vi "Rb_wavlength_lock.vi"(4 "Device":refnum<visa-resource-name>="GPIB0::10::INSTR", 6 "Settings":T2={"Module"=enum."WV Online TEC", "WV Online TEC"=23.169499999999484, "WV Online LD"=0.175, "WV Offline TEC"=29.51225, "WV Offline LD"=0.175, "WV Etalon TEC"=30.4, "HSRL Etalon TEC"=25.954, "HSRL TEC"=14.28699999999974, "HSRL LD"=0.16} {"HSRL LD" min=0.0 max=0.18 step=0.001 format="%.3p"; "HSRL TEC" min=14.0 max=28.0 step=0.1 format="%.3g"; "WV Offline LD" min=0.0 max=0.18 step=0.001 format="%.3p"; "WV Online LD" min=0.0 max=0.18 step=0.001 format="%.3p"; "HSRL Etalon TEC" format="%.2g"; "WV Etalon TEC" format="%.2g"; "WV Offline TEC" min=16.0 max=30.0 step=0.1 format="%.3g"; "WV Online TEC" min=14.0 max=28.0 step=0.1 format="%.3g"}, 7 "Lambda Set (nm)":dbl=828.198 format="%.5f", 8 "step_size":dbl=0.0005 format="%#_6p") -> (1 "Wavelength Lock":bool=TRUE, 2 "Lambda Read (nm)":dbl=828.197992104015 format="%.5f")   [LabVIEW 2012]
uses:
  <vilib>/DAQmx/write.llb/DAQmx Write (Digital 1D Bool NChan 1Samp 1Line).vi
  <vilib>/DAQmx/miscellaneous.llb/DAQmx Fill In Error Info.vi
  Shared Telescope WV DIAL Code/bristol/CLDevIFace.dll
panel:
  out "Readings":T1={"Pro8000"=TRUE, "WV OnLine TEC"=23.1755314, "WV Online TEC"=TRUE, "WV Online LD"=0.175443366, "WV Online LD"=TRUE, "WV Offline TEC"=29.5255375, "WV Offline TEC"=TRUE, "WV Offline LD"=0.175283208, "WV Offline LD"=TRUE, "WV EtalonTEC"=30.4229469, "WV Etalon TEC"=TRUE, "HSRL Etalon TEC"=25.9482574, "HSRL Etalon TEC"=TRUE, "HSRL TEC"=14.2977543, "HSRL TEC "=TRUE, "HSRL LD"=0.160093755, "HSRL LD"=TRUE} {"HSRL LD" format="%.3p"; "HSRL TEC" format="%.3g"; "WV Offline LD" format="%.3p"; "WV Online LD" format="%.3p"; "HSRL Etalon TEC" format="%.3g"; "WV EtalonTEC" format="%.3g"; "WV Offline TEC" format="%.3g"; "WV OnLine TEC" format="%.3g"}
  in  "Wavelength_lock_Tol":dbl=0.0001 format="%#_15g"
  out "WL_Difference":dbl=-7.895984936112654e-06 format="%#_3e"
  in  "Cancel lock":bool
  in  "Bristol In":i32=5
  out "Bristol Out":i32
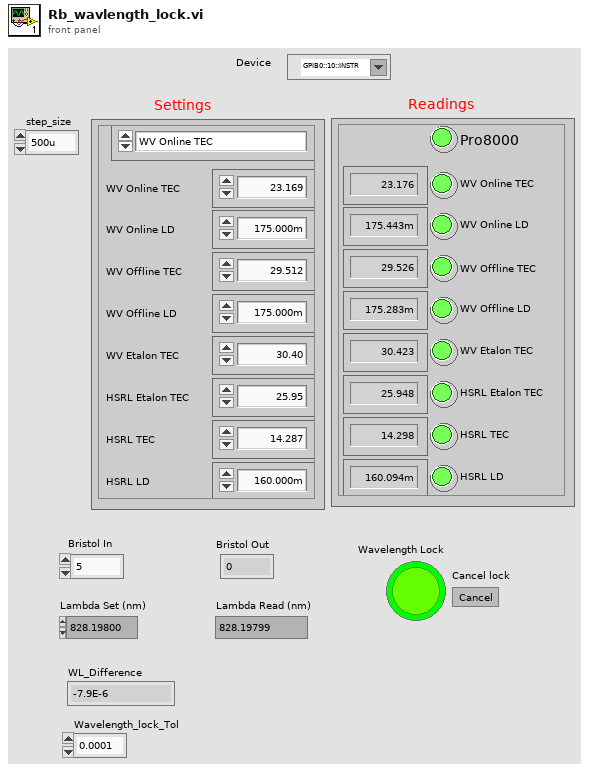
[diagram p1: front panel]
types:
  T1 = cluster{"Pro8000":bool, "WV OnLine TEC":dbl, "WV Online TEC":bool, "WV Online LD":dbl, "WV Online LD":bool, "WV Offline TEC":dbl, "WV Offline TEC":bool, "WV Offline LD":dbl, "WV Offline LD":bool, "WV EtalonTEC":dbl, "WV Etalon TEC":bool, "HSRL Etalon TEC":dbl, "HSRL Etalon TEC":bool, "HSRL TEC":dbl, "HSRL TEC ":bool, "HSRL LD":dbl, "HSRL LD":bool}
  T2 = cluster{"Module":enum16{"WV Online TEC", "WV Online LD", "WV Offline TEC", "WV Offline LD", "WV Etalon TEC", "HSRL Etalon TEC", "HSRL TEC", "HSRL LD"}, "WV Online TEC":dbl, "WV Online LD":dbl, "WV Offline TEC":dbl, "WV Offline LD":dbl, "WV Etalon TEC":dbl, "HSRL Etalon TEC":dbl, "HSRL TEC":dbl, "HSRL LD":dbl}
  T3 = enum16{"WV Online TEC", "WV Online LD", "WV Offline TEC", "WV Offline LD", "WV Etalon TEC", "HSRL Etalon TEC", "HSRL TEC", "HSRL LD"}
  T4 = enum16{"Open_TL", "Close_TL", "Verify_ID", "TEC_Sensor", "SET", "READ", "ON", "OFF", "Set_Limits", "Read_Limits", "Enable_Status", "Read_Status"}
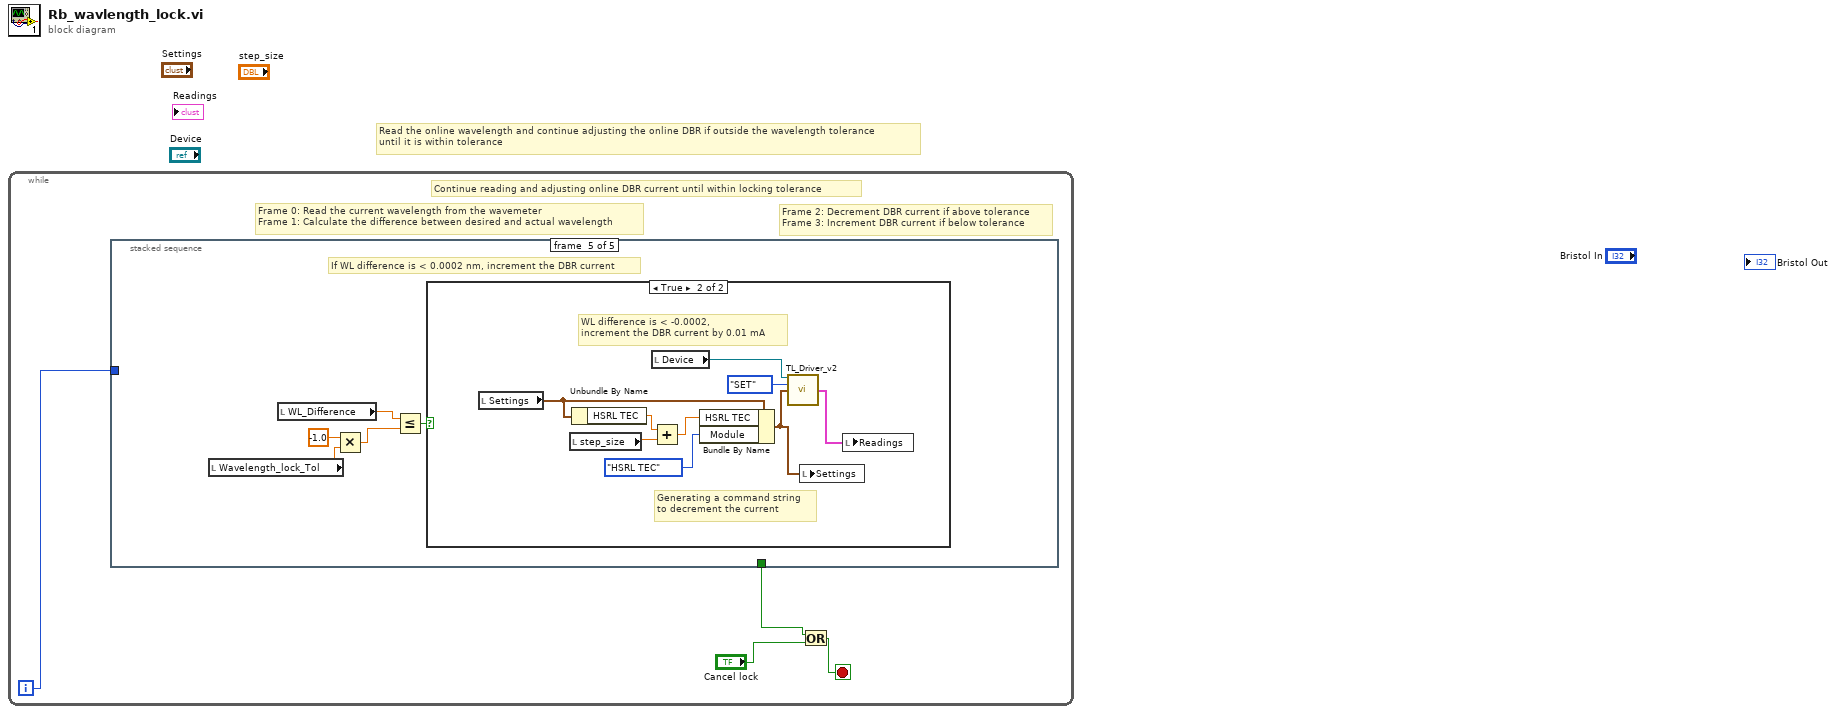
[diagram p0: block diagram]
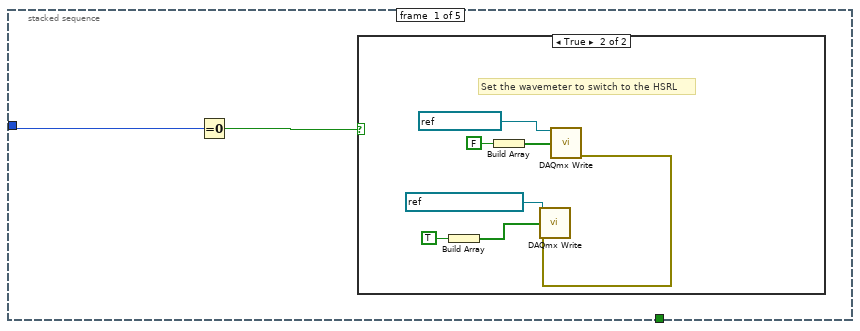
[diagram p2: hidden frame]
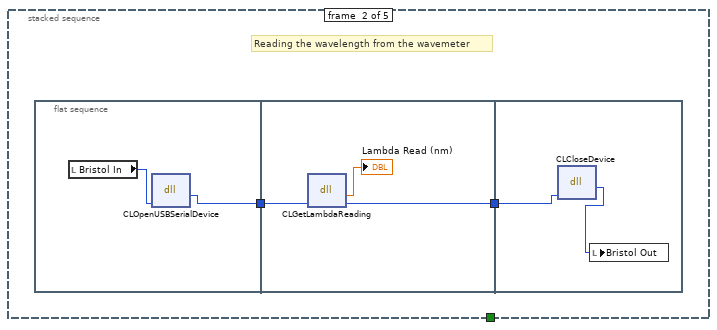
[diagram p4: hidden frame]
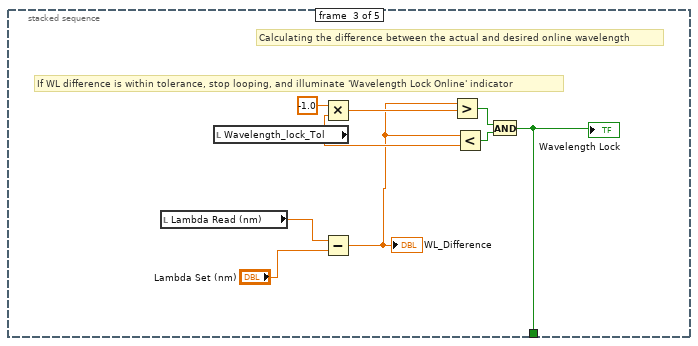
[diagram p5: hidden frame]
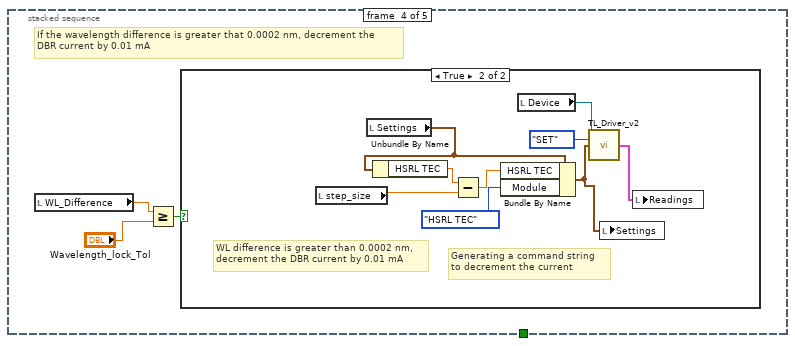
[diagram p6: hidden frame]
diagram:
  # "Read the online wavelength and continue adjusting the online DBR if outside the wavelength tolerance\nuntil it is within tolerance"
  n1 = while {
    i -> [w4]
    stop <- w1 stop-if-true
    # "Frame 2: Decrement DBR current if above tolerance\nFrame 3: Increment DBR current if below tolerance"
    # "Frame 0: Read the current wavelength from the wavemeter\nFrame 1: Calculate the difference between desired and actual wavelength"
    # "Continue reading and adjusting online DBR current until within locking tolerance"
    n2 = stacked-sequence {
      tunnel: w4 -> [w6 _ _ _ _]
      tunnel: [_ _ w23 _ _] -> w2
      frame #0 {
        n3 = Equal To 0?(x=w6) -> (x = 0?=w5:bool)
        n4 = case shown="True" w5 {
          frame False {
          }
          frame True {
            # "Set the wavemeter to switch to the HSRL"
            n5 = Build Array(TRUE ("Boolean")) -> (w8:bool[])
            n6 = Build Array(FALSE ("Boolean")) -> (w11:bool[])
            n7 = call-poly <vilib>:"DAQmx Write.vi"("task/channels in"=refnum<k21> "BristolWM", "data"=w11) -> ("error out"=w7:errorcluster)  [unwired: 11 in, 2 out]
            n8 = call-poly <vilib>:"DAQmx Write.vi"("task/channels in"=refnum<k21> "HSRL_WV_switch", "data"=w8, "error in"=w7) -> ()  [unwired: 10 in, 3 out]
          }
        }
      }
      frame #1 {
        # "Reading the wavelength from the wavemeter"
        n9 = flat-sequence {
          tunnel: [w16] -> w15
          tunnel: w15 -> [w19]
          tunnel: [w18] -> w14
          tunnel: w14 -> [w22]
          frame #0 {
            n10 = local read "Bristol In"() -> (w17:i32)
            n11 = dll-call lib="C:/Users/H2ODial/Desktop/Shared Telescope WV DIAL Code/bristol/CLDevIface.dll" fn="CLOpenUSBSerialDevice"("commPort"=w17) -> ("return type"=w16:i32)  [unwired: 4 in, 2 out]
          }
          frame #1 {
            n12 = dll-call lib="C:/Users/H2ODial/Desktop/Shared Telescope WV DIAL Code/bristol/CLDevIface.dll" fn="CLGetLambdaReading"("devHandle"=w19) -> ("return type"=→"Lambda Read (nm)":dbl, "devHandle"=w18:i32)  [unwired: 3 in, 2 out]
          }
          frame #2 {
            n13 = dll-call lib="C:/Users/H2ODial/Desktop/Shared Telescope WV DIAL Code/bristol/CLDevIface.dll" fn="CLCloseDevice"("commPort"=w22) -> ("return type"=w21:i32)  [unwired: 4 in, 2 out]
            n14 = local write "Bristol Out"(w21) -> ()
          }
        }
      }
      frame #2 {
        # "If WL difference is within tolerance, stop looping, and illuminate 'Wavelength Lock Online' indicator"
        # "Calculating the difference between the actual and desired online wavelength"
        n15 = local read "Lambda Read (nm)"() -> (w31:dbl)
        n16 = local read "Wavelength_lock_Tol"() -> (w28:dbl)
        n17 = Multiply(x=-1.0, y=w28) -> (x*y=w29:dbl)
        n18 = Subtract(x=w31, y="Lambda Set (nm)") -> (x-y=w24:dbl)
        "WL_Difference" <- w24
        n19 = Greater?(x=w24, y=w29) -> (0:w25:bool)
        n20 = Less?(x=w24, y=w28) -> (x < y?=w26:bool)
        n21 = And(x=w25, y=w26) -> (x .and. y?=w23:bool)
        "Wavelength Lock" <- w23
      }
      frame #3 {
        # "If the wavelength difference is greater that 0.0002 nm, decrement the \nDBR current by 0.01 mA"
        n22 = local read "WL_Difference"() -> (w34:dbl)
        n23 = Greater Or Equal?(x=w34, y="Wavelength_lock_Tol") -> (x >= y?=w33:bool)
        n24 = case shown="True" w33 {
          frame False {
            # "Wavelength difference is not greater than 0.0002 nm, do nothing"
          }
          frame True {
            # "Generating a command string\nto decrement the current"
            # "WL difference is greater than 0.0002 nm,\ndecrement the DBR current by 0.01 mA"
            n25 = local read "step_size"() -> (w40:dbl)
            n26 = local read "Settings"() -> (w39:T2)
            n27 = Unbundle By Name(w39) -> ("HSRL TEC"=w43:dbl)
            n28 = Subtract(x=w43, y=w40) -> (x-y=w42:dbl)
            n29 = Bundle By Name(cluster=w39, "HSRL TEC"=w42, "Module"=T3."HSRL TEC") -> (w35:T2)
            n30 = local read "Device"() -> (w38:refnum<visa-resource-name>)
            n31 = call "TL_Driver_v2.vi"("Device In"=w38, "Commands"=T4."SET", "Settings"=w35) -> ("Readings"=w37:T1)  [unwired: 9 in, 3 out]
            n32 = local write "Settings"(w35) -> ()
            n33 = local write "Readings"(w37) -> ()
          }
        }
      }
      frame #4 {
        # "If WL difference is < 0.0002 nm, increment the DBR current"
        n34 = local read "Wavelength_lock_Tol"() -> (w45:dbl)
        n35 = local read "WL_Difference"() -> (w48:dbl)
        n36 = Multiply(x=-1.0, y=w45) -> (x*y=w44:dbl)
        n37 = Less Or Equal?(x=w48, y=w44) -> (x <= y?=w47:bool)
        n38 = case shown="True" w47 {
          frame False {
            # "WL difference is no <= to -0.0002 nm, do nothing"
          }
          frame True {
            # "WL difference is < -0.0002,\nincrement the DBR current by 0.01 mA"
            # "Generating a command string\nto decrement the current"
            n39 = local read "Settings"() -> (w57:T2)
            n40 = local read "step_size"() -> (w52:dbl)
            n41 = Unbundle By Name(w57) -> ("HSRL TEC"=w56:dbl)
            n42 = local read "Device"() -> (w53:refnum<visa-resource-name>)
            n43 = Add(x=w56, y=w52) -> (x+y=w55:dbl)
            n44 = Bundle By Name(cluster=w57, "HSRL TEC"=w55, "Module"=T3."HSRL TEC") -> (w49:T2)
            n45 = call "TL_Driver_v2.vi"("Device In"=w53, "Commands"=T4."SET", "Settings"=w49) -> ("Readings"=w50:T1)  [unwired: 9 in, 3 out]
            n46 = local write "Settings"(w49) -> ()
            n47 = local write "Readings"(w50) -> ()
          }
        }
      }
    }
    n48 = Or(x=w2, y="Cancel lock") -> (x .or. y?=w1:bool)
  }
